vi "json_cache.vi"(7 "action":enum8{"null", "get", "create", "delete"}(ring), 8 "error in (no error)":errorcluster, 10 "cache id in":u64, 11 "elements in":T1[](array[typedef])) -> (0 "error out":errorcluster, 1 "exists?":bool, 2 "cache id out":u64, 3 "elements out":T1[](array[typedef]), 5 "cache ids":u64[](array[numeric]))   [LabVIEW 2017]
uses:
  json_element.ctl
  json_element_type.ctl
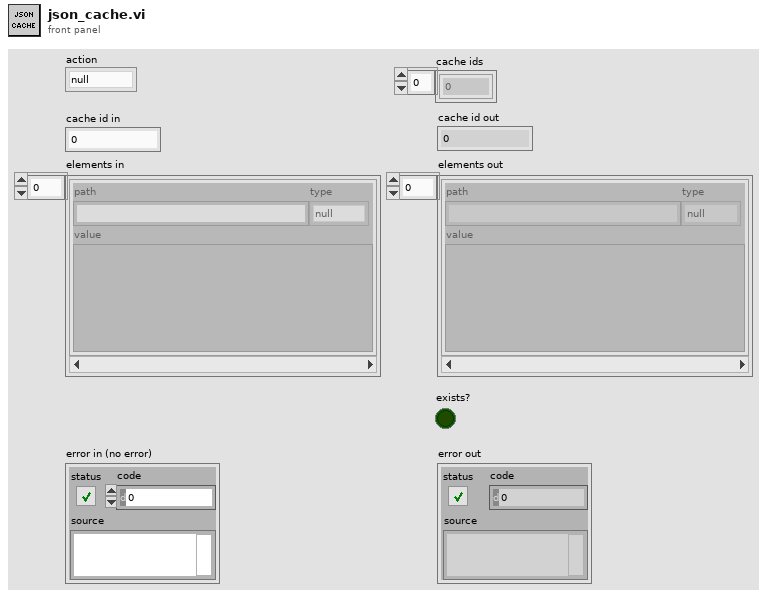
[diagram p1: front panel]
types:
  T1 = typedef "json_element.ctl" = cluster{"path":string, "type":T2, "value":variant}
  T2 = typedef "json_element_type.ctl" = enum8{"null", "bool", "int", "uint", "float", "string", "array", "object"}
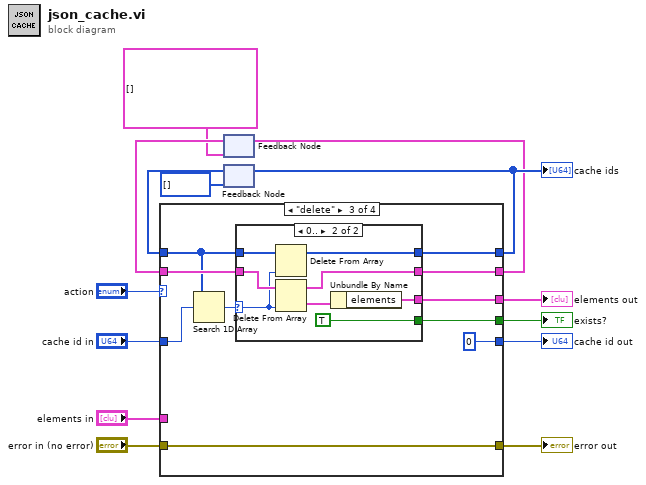
[diagram p0: block diagram]
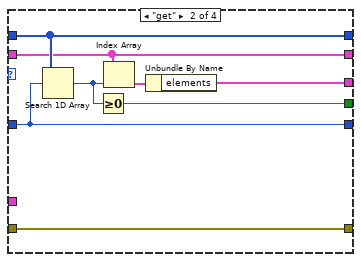
[diagram p3: hidden frame]
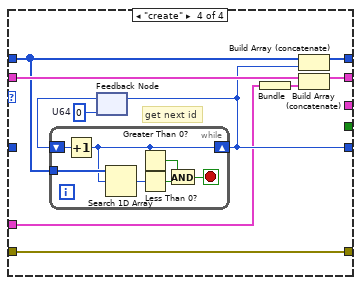
[diagram p5: hidden frame]
diagram:
  n1 = feedback #1(cluster{"elements":T1[]}[] [] ("cache")) -> (w9:cluster{"elements":T1[]}[])
  n2 = feedback #2(u64[] []) -> (w11:u64[])
  n3 = case shown="\"delete\"" "action" {
    tunnel: [w17 w26 w31 w50] -> w12
    tunnel: w11 -> [w17 w26 w32 w52]
    tunnel: [w16 w25 w33 w51] -> w10
    tunnel: w9 -> [w16 w25 w34 w56]
    tunnel: "cache id in" -> [w15 w21 w36 _]
    tunnel: [_ w22 w27 _] -> w6
    tunnel: [w15 w21 u64 0 ("U64") w49] -> w5
    tunnel: [_ w20 w29 _] -> w4
    tunnel: [w18 w19 w35 w55] -> w3
    tunnel: "error in (no error)" -> [w18 w19 w35 w55]
    tunnel: "elements in" -> [_ _ _ w47]
    frame "null" {
    }
    frame "get" {
      n4 = Search 1D Array(1D array=w26, element=w21) -> (index of element=w24:i32)  [unwired: 1 in]
      n5 = Greater Or Equal To 0?(x=w24) -> (x >= 0?=w20:bool)
      n6 = Index Array(array=w25, index=w24) -> (element=w23:cluster{"elements":T1[]})
      n7 = Unbundle By Name(w23) -> ("elements"=w22:T1[])
    }
    frame "delete" {
      n8 = Search 1D Array(1D array=w32, element=w36) -> (index of element=w30:i32)  [unwired: 1 in]
      n9 = case shown="0.." w30 {
        selector: w30 -> [_ w42]
        tunnel: w34 -> [w37 w46]
        tunnel: [w37 w45] -> w33
        tunnel: w32 -> [w38 w44]
        tunnel: [w38 w43] -> w31
        tunnel: [_ TRUE] -> w29
        tunnel: [_ w39] -> w27
        frame ..-1 {
        }
        frame 0.. {
          n10 = Delete From Array(array=w44, index=w42) -> (array with subset deleted=w43:u64[])  [unwired: 1 in, 1 out]
          n11 = Delete From Array(array=w46, index=w42) -> (deleted portion=w40:cluster{"elements":T1[]}, array with subset deleted=w45:cluster{"elements":T1[]}[])  [unwired: 1 in]
          n12 = Unbundle By Name(w40) -> ("elements"=w39:T1[])
        }
      }
    }
    frame "create" {
      w54 = u64 0  # U64
      # "get next id"
      n13 = feedback #3(w54) -> (w53:u64)
      n14 = while {
        shift-right: [w60] -> w49
        shift-left: w53 -> [w63]
        tunnel: w52 -> [w62]
        stop <- w57 stop-if-true
        n15 = Increment(x=w63) -> (x+1=w60:u64)
        n16 = Search 1D Array(1D array=w62, element=w60) -> (index of element=w61:i32)  [unwired: 1 in]
        n17 = Greater Than 0?(x=w60) -> (x > 0?=w58:bool)
        n18 = Less Than 0?(x=w61) -> (x < 0?=w59:bool)
        n19 = And(x=w58, y=w59) -> (x .and. y?=w57:bool)
      }
      n20 = feedback-in #3(w49) -> ()
      n21 = Bundle("elements in"=w47) -> (w48:cluster{"elements in":T1[]})  [unwired: 1 in]
      n22 = Build Array (concatenate)(w52, w49) -> (w50:u64[])
      n23 = Build Array (concatenate)(w56, w48) -> (w51:cluster{"elements in":T1[]}[])
    }
  }
  "error out" <- w3
  "elements out" <- w6
  "cache id out" <- w5
  "exists?" <- w4
  "cache ids" <- w12
  n24 = feedback-in #1(w10) -> ()
  n25 = feedback-in #2(w12) -> ()
